vi "Set Index.vi"(8 "error in (no error)":errorcluster, 10 "Index":u16, 11 "OD Entry in":refnum<class "OD Entry.lvclass">) -> (0 "error out":errorcluster, 3 "OD Entry out":refnum<class "OD Entry.lvclass">)   [LabVIEW 2024, in "OD Entry.lvclass"]
uses:
  OD Entry.lvclass
  OD Entry.lvclass/OD Entry.ctl
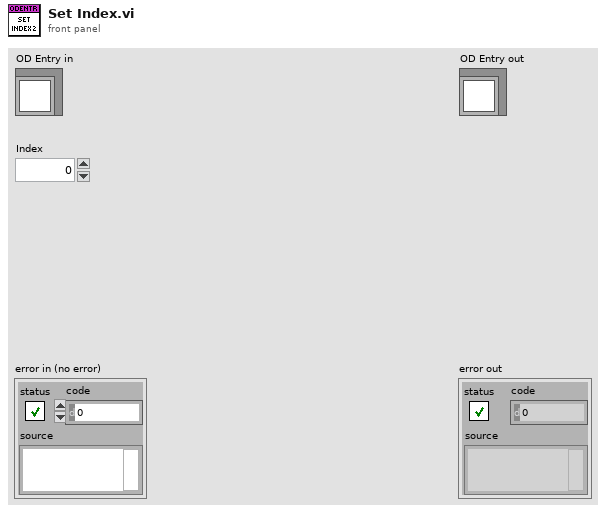
[diagram p1: front panel]
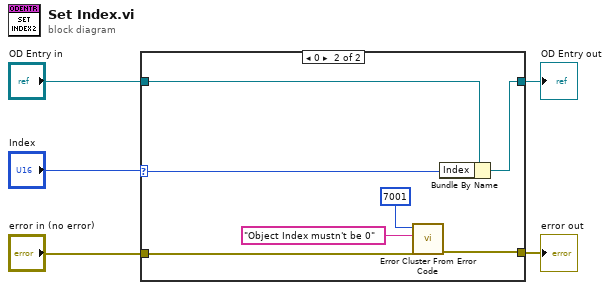
[diagram p0: block diagram]
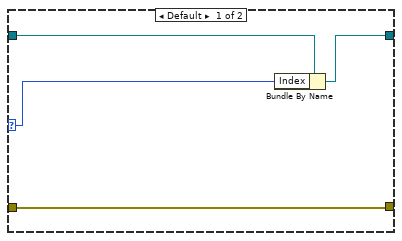
[diagram p2: hidden frame]
diagram:
  n1 = case shown="0" "Index" {
    selector: "Index" -> [w6 w14]
    tunnel: "OD Entry in" -> [w9 w16]
    tunnel: [w8 w15] -> w4
    tunnel: "error in (no error)" -> [w7 w11]
    tunnel: [w7 w10] -> w1
    frame Default {
      n2 = Bundle By Name(cluster=w9, "Index"=w6) -> (w8:refnum<class "OD Entry.lvclass">)
    }
    frame 0 {
      n3 = call <vilib>:"Error Cluster From Error Code.vi"("error in (no error)"=w11, "error message (\"\")"="Object Index mustn't be 0" ("error message (\"\")"), "error code (0)"=7001) -> ("error out"=w10:errorcluster)  [unwired: 6 in]
      n4 = Bundle By Name(cluster=w16, "Index"=w14) -> (w15:refnum<class "OD Entry.lvclass">)
    }
  }
  "error out" <- w1
  "OD Entry out" <- w4
